vi "RT_Control_Adrian_AllIncluded.vi"(10 "rt fifo":refnum<k33>, 11 "Parameters":T1) -> (0 "error out":errorcluster, 2 "Delayed Cycles":dbl)   [LabVIEW 2021]
uses:
  parametersRT.ctl
  <vilib>/DAQmx/write.llb/DAQmx Write (Analog 1D DBL NChan 1Samp).vi
  <vilib>/DAQmx/read.llb/DAQmx Read (Analog 1D DBL NChan 1Samp).vi
  <vilib>/DAQmx/read.llb/DAQmx Read (Digital 2D U32 NChan NSamp).vi
  <vilib>/Analysis/baseanly.llb/Mean (DBL).vi
  <vilib>/DAQmx/configure/timing.llb/DAQmx Timing (Sample Clock).vi
  <vilib>/DAQmx/miscellaneous.llb/DAQmx Fill In Error Info.vi
  <resource>/objmgr/daqmx.rc
  <vilib>/Analysis/NI_AALBase.lvlib
panel:
  out "error out 7":errorcluster
  out "error out 6":errorcluster
  out "error out 5":errorcluster
  out "error out 4":errorcluster
  out "error out 3":errorcluster
  out "error out 2":errorcluster
  out "FB Raw Readings":dbl[][](array[numeric])
  in  "Stop Loop":bool
  in  "System Information":enum32{"RT System"}(tab)
  in  "source":tag
  in  "source 2":tag
  in  "RT Data Monitoring":enum32{"Forces", "Angles", "Power", "Pressure"}(tab)
  out "Bias Voltages":dbl[][](array[numeric])=[[-0.0710179470114859, -0.17463349299050945, -0.11016159714741332, 0.026018829634351103, 0.12897648926553976, 0.08259620236774425]]
  out "Bias Vector":dbl[](array[numeric])=[-0.0710179470114859, -0.17463349299050945, -0.11016159714741332, 0.026018829634351103, 0.12897648926553976, 0.08259620236774425]
  in  "Bias":bool
  in  "Unbias":bool
  in  "Zero Angle  Offset":dbl[](array[numeric])=[8.53, -8.09, 79.37, 29.36]
  # "Important! Set angle offset before reading angles"
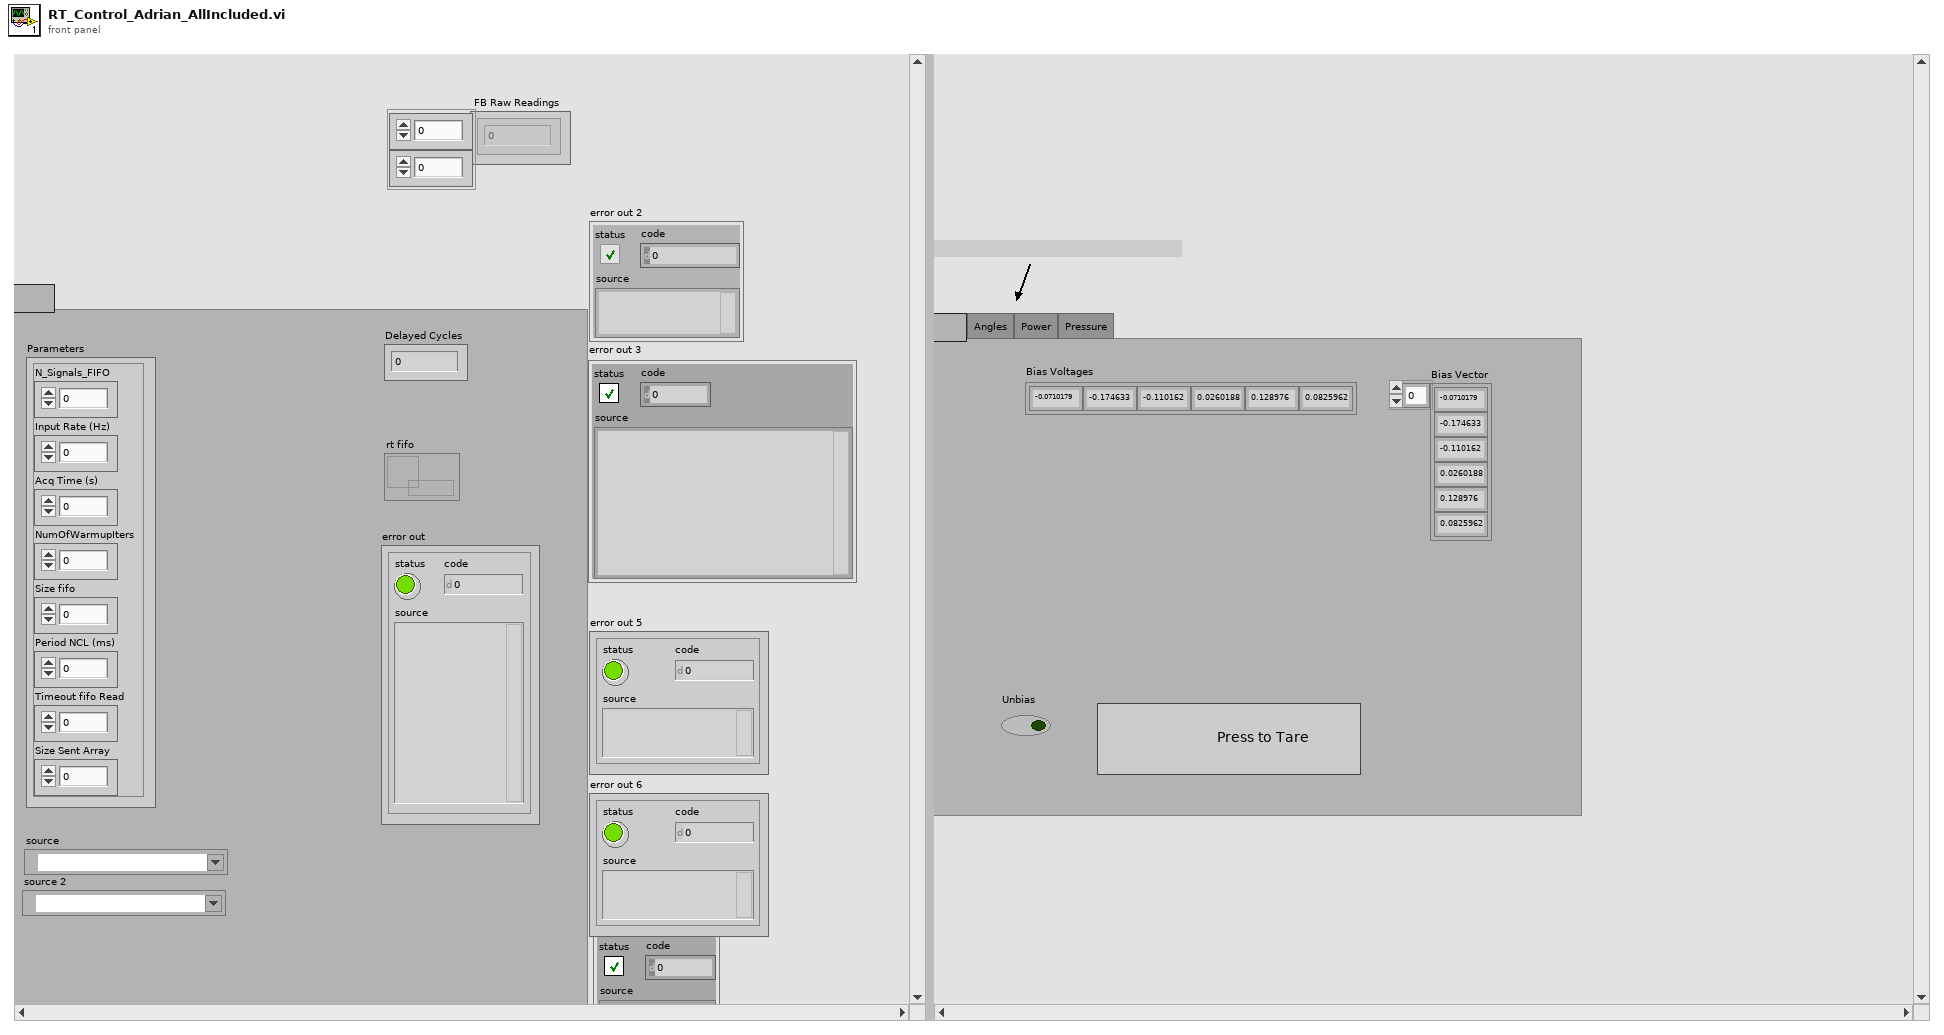
[diagram p1: front panel]
types:
  T1 = typedef "parametersRT.ctl" = cluster{"N_Signals_FIFO":u32, "Input Rate (Hz)":dbl, "Acq Time (s)":dbl, "NumOfWarmupIters":u32, "Size fifo":u32, "Period NCL (ms)":i64, "Timeout fifo Read":i32, "Size Sent Array":i32}
  T2 = cluster{"Csn task out":refnum<k21>, "CLK task out":refnum<k21>, "D0 task out":refnum<k21>}
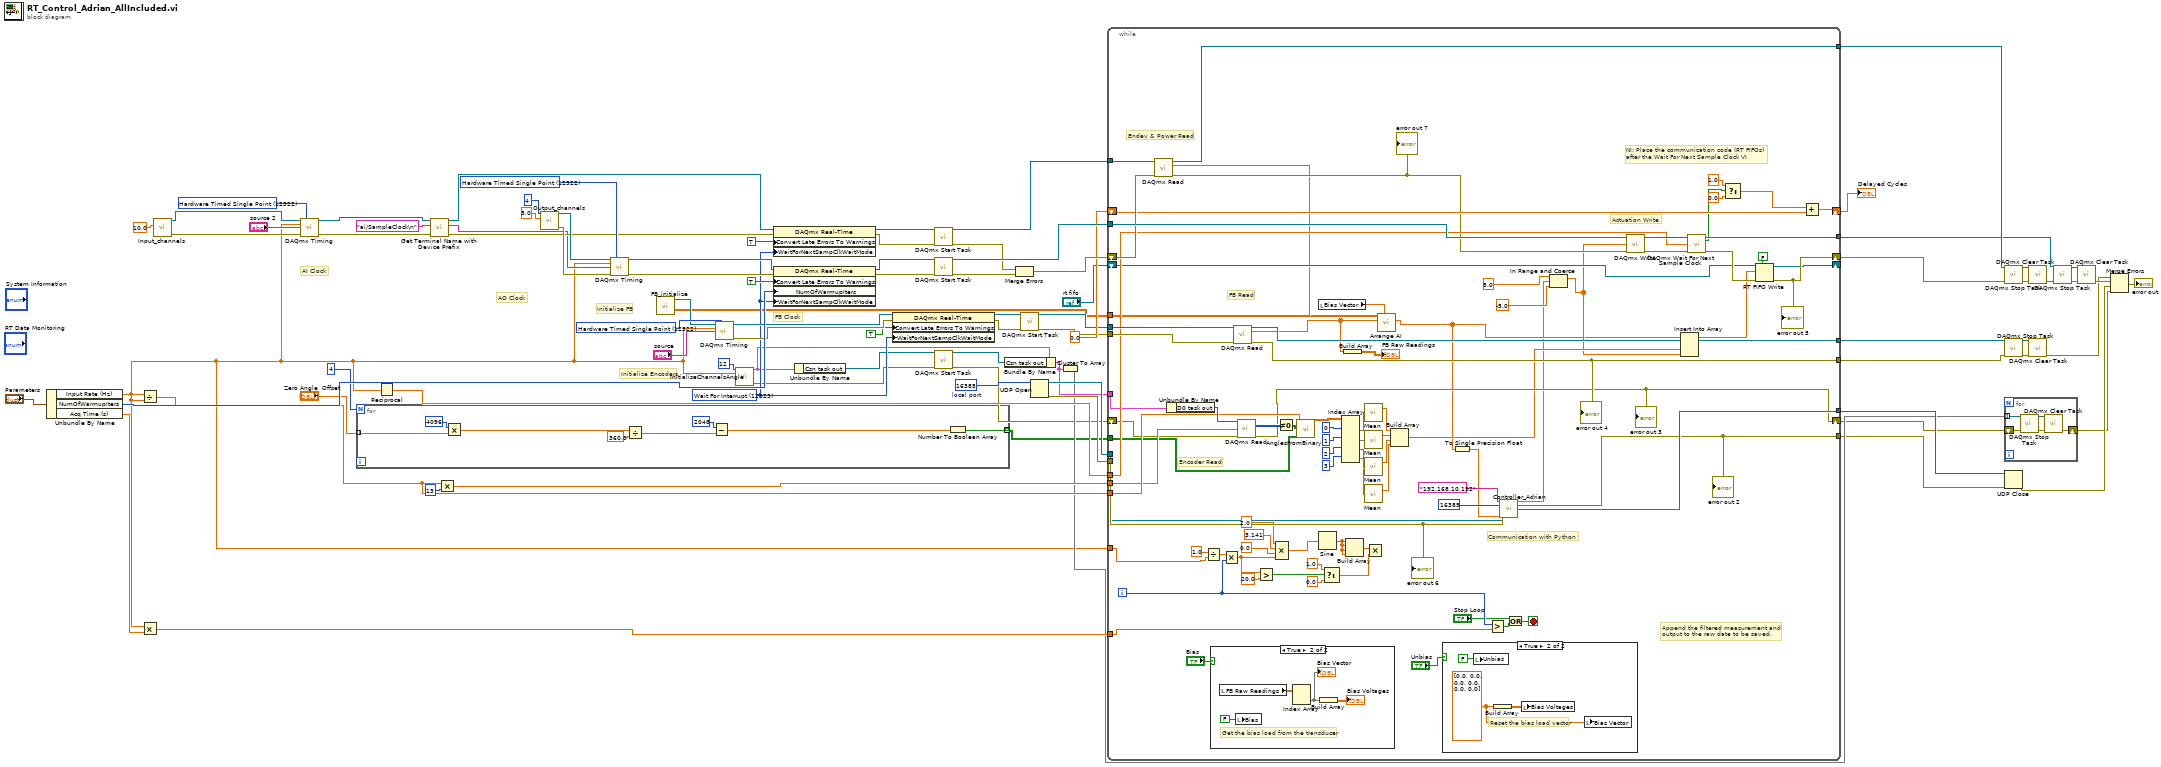
[diagram p0: block diagram]
diagram:
  w49 = 12522 items=["Finite Samples"=10178, "Continuous Samples"=10123, "Hardware Timed Single Point"=12522] ("sample mode")
  w59 = u16 16385  # local port
  w66 = 12522 items=["Finite Samples"=10178, "Continuous Samples"=10123, "Hardware Timed Single Point"=12522] ("sample mode")
  w44 = 12523 items=["Wait For Interrupt"=12523, "Poll"=12524, "Yield"=12525] ("WaitForNextSampClkWaitMode")
  w86 = 12522 items=["Finite Samples"=10178, "Continuous Samples"=10123, "Hardware Timed Single Point"=12522] ("sample mode")
  # "Initialize Encoders"
  # "Initialize FB"
  # "AO Clock"
  # "AI Clock"
  # "FB Clock"
  n1 = Unbundle By Name("Parameters") -> ("Input Rate (Hz)"=w1:dbl, "NumOfWarmupIters"=w73:u32, "Acq Time (s)"=w80:dbl)
  n2 = Divide(x=w1, y=w1) -> (x/y=w11:dbl)
  n3 = Multiply(x=w1, y=w80) -> (x*y=w54:dbl)
  n4 = call "Input_channels.vi"("Range"=10.0) -> ("error out"=w68:errorcluster, "Refnum out"=w67:refnum<k21>)  [unwired: 9 in]
  n5 = call-poly <vilib>:"DAQmx Timing.vi"("task/channels in"=w67, "sample mode"=w66, "rate"=w1, "source"="source 2", "error in"=w68) -> ("task out"=w37:refnum<k21>, "error out"=w35:errorcluster)  [unwired: 9 in]
  n6 = for {
    N: 4 -> [_]
    tunnel: [w91] -> w3 mode=indexing
    tunnel: "Zero Angle  Offset" -> [w94] mode=indexing
    n7 = Multiply(x=4096, y=w94) -> (x*y=w95:dbl)
    n8 = Divide(x=w95, y=360.0) -> (x/y=w89:dbl)
    n9 = Subtract(x=2048, y=w89) -> (x-y=w88:dbl)
    n10 = Number To Boolean Array(number=w88) -> (Boolean array=w91:bool[])
  }
  n11 = Reciprocal(x=w1) -> (1/x=w85:dbl)
  n12 = call "Get Terminal Name with Device Prefix.vi"("error in (no error)"=w35, "Local Terminal Name"="ai/SampleClock\n", "task/channels in"=w37) -> ("error out"=w34:errorcluster, "Terminal Name with Device Prefix"=w33:tag, "task out"=w36:refnum<k21>)  [unwired: 6 in]
  n13 = Multiply(x=w11, y=13) -> (x*y=w9:dbl)
  n14 = call "Output_channels.vi"("Range"=5.0 ("Maximum Value"), "nchan"=4) -> ("error out"=w77:errorcluster, "Refnum out"=w76:refnum<k21>)  [unwired: 8 in]
  n15 = call-poly <vilib>:"DAQmx Timing.vi"("task/channels in"=w76, "sample mode"=w86, "rate"=w1, "source"=w33, "error in"=w77) -> ("task out"=w84:refnum<k21>, "error out"=w83:errorcluster)  [unwired: 9 in]
  n16 = call "FB_initialize.vi"() -> ("Transformed Calibration Matrix"=w41:dbl[][], "FB out"=w45:refnum<k21>)  [unwired: 9 in, 1 out]
  n17 = call-poly <vilib>:"DAQmx Timing.vi"("task/channels in"=w45, "sample mode"=w49, "rate"=w1, "source"="source") -> ("task out"=w51:refnum<k21>, "error out"=w50:errorcluster)  [unwired: 10 in]
  n18 = call "InitialiseChannelsAngle.vi"("Number of data bits"=12, "Fs"=w1) -> ("output cluster"=w12:T2, "error out"=w13:errorcluster)  [unwired: 12 in]
  n19 = property class="DAQmx Real-Time"(reference=w36, error in=w34, "Convert Late Errors To Warnings"=TRUE, "WaitForNextSampClkWaitMode"=w44) -> (reference out=w63:refnum<k21>, error out=w62:errorcluster)
  n20 = property class="DAQmx Real-Time"(reference=w84, error in=w83, "Convert Late Errors To Warnings"=TRUE, "NumOfWarmupIters"=w73, "WaitForNextSampClkWaitMode"=w44) -> (reference out=w81:refnum<k21>, error out=w70:errorcluster)
  n21 = Unbundle By Name(w12) -> ("Csn task out"=w17:refnum<k21>)
  n22 = property class="DAQmx Real-Time"(reference=w51, error in=w50, "Convert Late Errors To Warnings"=TRUE ("ConvLateErrorsToWarnings"), "WaitForNextSampClkWaitMode"=w44) -> (reference out=w46:refnum<k21>, error out=w47:errorcluster)
  n23 = call <vilib>:"DAQmx Start Task.vi"("task/channels in"=w63, "error in"=w62) -> ("task out"=w79:refnum<k21>, "error out"=w61:errorcluster)  [unwired: 12 in]
  n24 = call <vilib>:"DAQmx Start Task.vi"("task/channels in"=w81, "error in"=w70) -> ("task out"=w78:refnum<k21>, "error out"=w69:errorcluster)  [unwired: 12 in]
  n25 = call <vilib>:"DAQmx Start Task.vi"("task/channels in"=w17, "error in"=w13) -> ("task out"=w16:refnum<k21>, "error out"=w6:errorcluster)  [unwired: 12 in]
  n26 = Bundle By Name(cluster=w12, "Csn task out"=w16) -> (w10:T2)
  n27 = Merge Errors(w61, w69) -> (w60:errorcluster)
  n28 = call <vilib>:"DAQmx Start Task.vi"("task/channels in"=w46, "error in"=w47) -> ("task out"=w43:refnum<k21>, "error out"=w42:errorcluster)  [unwired: 12 in]
  n29 = UDP Open(11:w59) -> (port=w57:refnum<k16>, 0:w58:errorcluster)  [unwired: 4 in, 1 out]
  n30 = Cluster To Array(cluster=w10) -> (array=w8:refnum<k21>[])
  n31 = while {
    shift-right: [w134] -> w26
    shift-left: w60 -> [w174]
    shift-right: [w179] -> w87
    shift-left: 0.0 ("f") -> [w168]
    tunnel: w85 -> [w157]
    tunnel: w54 -> [w178]
    tunnel: w78 -> [w177]
    tunnel: [w175] -> w25
    tunnel: w79 -> [w176]
    tunnel: [w159] -> w21
    tunnel: w58 -> [w173]
    tunnel: w57 -> [w172]
    tunnel: [w171] -> w56
    tunnel: w43 -> [w167]
    tunnel: w42 -> [w166]
    tunnel: w41 -> [w106]
    tunnel: [w163] -> w31
    tunnel: [w162] -> w29
    tunnel: w11 -> [w140]
    tunnel: w10 -> [w139]
    tunnel: w9 -> [w138]
    shift-right: [w137] -> w7
    shift-left: w6 -> [w136]
    shift-right: [w132] -> _
    shift-left: "rt fifo" -> [w131]
    tunnel: w3 -> [w114]
    tunnel: [w113] -> w2
    tunnel: w1 -> [w112]
    i -> [w125]
    stop <- w109 stop-if-true
    # "NI: Place the communication code (RT FIFOs) \nafter the Wait For Next Sample Clock VI"
    # "Communication with Python"
    # "Actuation Write"
    # "Encoder Read"
    # "Endev & Power Read"
    # "FB Read"
    # "Append the filtered measurement and \noutput to the raw date to be saved."
    n32 = call-poly <vilib>:"DAQmx Read.vi"("task/channels in"=w176, "error in"=w174) -> ("task out"=w175:refnum<k21>, "data"=w108:dbl[], "error out"=w129:errorcluster)  [unwired: 11 in]
    "error out 7" <- w129
    n33 = Unbundle By Name(w139) -> ("D0 task out"=w156:refnum<k21>)
    n34 = Divide(x=1.0, y=w112) -> (x/y=w123:dbl)
    n35 = case shown="True" "Bias" {
      frame False {
      }
      frame True {
        # "Get the bias load from the transducer"
        n36 = local read "FB Raw Readings"() -> (w189:dbl[][])
        n37 = local write "Bias"(FALSE) -> ()
        n38 = Index Array(array=w189) -> (element=w186:dbl[])  [unwired: 2 in]
        "Bias Vector" <- w186
        n39 = Build Array(w186) -> (→"Bias Voltages":dbl[][])
      }
    }
    n40 = Multiply(x=w123, y=w125) -> (x*y=w119:dbl)
    n41 = call-poly <vilib>:"DAQmx Read.vi"("task/channels in"=w167, "error in"=w166) -> ("task out"=w163:refnum<k21>, "data"=w103:dbl[], "error out"=w162:errorcluster)  [unwired: 11 in]
    "error out 4" <- w162
    n42 = call-poly <vilib>:"DAQmx Read.vi"("task/channels in"=w156, "number of samples per channel"=w138, "error in"=w136) -> ("data"=w155:u32[][], "error out"=w137:errorcluster)  [unwired: 10 in, 1 out]
    "error out 3" <- w137
    n43 = Greater?(x=w119, y=20.0) -> (0:w115:bool)
    n44 = Compound Arithmetic op=MULTIPLY(2.0 ("value"), 3.141 ("value"), 0.0 ("value"), w119) -> (w122:dbl)
    n45 = Not Equal To 0?(x=w155) -> (x != 0?=w141:bool[][])
    n46 = call "AnglesFromBinary.vi"("Binary Offset"=w114, "Array"=w141, "Buffer Length"=w140) -> ("Unwrapped Phase"=w154:dbl[][])  [unwired: 8 in]
    n47 = local read "Bias Vector"() -> (w107:dbl[])
    n48 = Sine(x=w122) -> (sin(x)=w121:dbl)
    n49 = Select(t=1.0, s=w115, f=0.0) -> (s? t:f=w105:dbl)
    n50 = Index Array(array=w154, index (row) #1=0 ("index (row)"), index (row) #2=1 ("index (row)"), index (row) #3=2 ("index (row)"), index (row) #4=3 ("index (row)")) -> (element #1=w149:dbl[], element #2=w148:dbl[], element #3=w147:dbl[], element #4=w146:dbl[])  [unwired: 4 in]
    n51 = Build Array(w103) -> (→"FB Raw Readings":dbl[][])
    n52 = Build Array(w121, w121, w121, w121) -> (w120:dbl[])
    n53 = call-poly <vilib>:"Mean.vi"("X"=w149) -> ("mean"=w142:dbl)  [unwired: 1 out]
    n54 = call-poly <vilib>:"Mean.vi"("X"=w148) -> ("mean"=w143:dbl)  [unwired: 1 out]
    n55 = call-poly <vilib>:"Mean.vi"("X"=w147) -> ("mean"=w144:dbl)  [unwired: 1 out]
    n56 = call-poly <vilib>:"Mean.vi"("X"=w146) -> ("mean"=w145:dbl)  [unwired: 1 out]
    n57 = Multiply(x=w120, y=w105) -> ()  [unwired: 1 out]
    n58 = call "Arrange AI.vi"("Transformed Calibration Matrix"=w106, "Bias Vector"=w107, "FB data"=w103, "EDV + Voltage data"=w108) -> ("FIFO Data (7EDV+3Force+4Power+4Voltage)"=w97:dbl[])  [unwired: 6 in, 1 out]
    n59 = Build Array(w142, w143, w144, w145) -> (w104:dbl[])
    n60 = case shown="True" "Unbias" {
      frame False {
      }
      frame True {
        w184 = dbl[] [0.0, 0.0, 0.0, 0.0, 0.0, 0.0]
        # "Reset the bias load vector"
        n61 = local write "Unbias"(FALSE) -> ()
        n62 = Build Array(w184) -> (w183:dbl[][])
        n63 = local write "Bias Voltages"(w183) -> ()
        n64 = local write "Bias Vector"(w184) -> ()
      }
    }
    n65 = To Single Precision Float(number=w97) -> (single precision float=w98:sgl[])
    n66 = Greater?(x=w125, y=w178) -> (0:w110:bool)
    n67 = call "Controller_Adrian.vi"("name 2"="192.168.10.192", "port or service name"=u16 16389, "connection ID"=w172, "error in (no error)"=w173, "x"=w98) -> ("*(type *) &x"=w96:dbl[], "error out"=w113:errorcluster, "connection ID out"=w171:refnum<k16>)  [unwired: 8 in]
    "error out 2" <- w113
    n68 = Or(x="Stop Loop", y=w110) -> (x .or. y?=w109:bool)
    n69 = In Range and Coerce(upper limit=5.0, x=w96, lower limit=-5.0) -> (coerced(x)=w101:dbl[])  [unwired: 1 out]
    n70 = call-poly <vilib>:"DAQmx Write.vi"("task/channels in"=w177, "data"=w101, "error in"=w129) -> ("task out"=w160:refnum<k21>, "error out"=w161:errorcluster)  [unwired: 10 in, 1 out]
    n71 = Insert Into Array(array=w97, new element #1=w104, new element #2=w101) -> (w130:dbl[])  [unwired: 1 in]
    n72 = call <vilib>:"DAQmx Wait For Next Sample Clock.vi"("task/channels in"=w160, "timeout (sec)"=w157, "error in"=w161) -> ("task out"=w159:refnum<k21>, "is late?"=w158:bool, "error out"=w133:errorcluster)  [unwired: 10 in]
    n73 = Select(t=1.0, s=w158, f=0.0) -> (s? t:f=w180:dbl)
    n74 = RT FIFO Write(0:w131, 1:w130, 3:w133, 5:FALSE ("overwrite on timeout (T)")) -> (8:w132:refnum<k33>, 11:w134:errorcluster)  [unwired: 1 in, 2 out]
    "error out 5" <- w134
    n75 = Add(x=w180, y=w168) -> (x+y=w179:dbl)
    "error out 6" <- w173
  }
  "Delayed Cycles" <- w87
  n76 = call <vilib>:"DAQmx Stop Task.vi"("task/channels in"=w25, "error in"=w26) -> ("task out"=w24:refnum<k21>, "error out"=w27:errorcluster)  [unwired: 12 in]
  n77 = call <vilib>:"DAQmx Stop Task.vi"("task/channels in"=w31, "error in"=w29) -> ("task out"=w30:refnum<k21>, "error out"=w28:errorcluster)  [unwired: 12 in]
  n78 = for {
    tunnel: w8 -> [w194] mode=indexing
    shift-right: [w190] -> w5
    shift-left: w7 -> [w192]
    n79 = call <vilib>:"DAQmx Stop Task.vi"("task/channels in"=w194, "error in"=w192) -> ("task out"=w193:refnum<k21>, "error out"=w191:errorcluster)  [unwired: 12 in]
    n80 = call <vilib>:"DAQmx Clear Task.vi"("task in"=w193, "error in"=w191) -> ("error out"=w190:errorcluster)  [unwired: 13 in]
  }
  n81 = UDP Close(connection ID=w56, 8:w2) -> (error out=w55:errorcluster)  [unwired: 1 out]
  n82 = call <vilib>:"DAQmx Clear Task.vi"("task in"=w24, "error in"=w27) -> ("error out"=w23:errorcluster)  [unwired: 13 in]
  n83 = call <vilib>:"DAQmx Clear Task.vi"("task in"=w30, "error in"=w28) -> ("error out"=w40:errorcluster)  [unwired: 13 in]
  n84 = call <vilib>:"DAQmx Stop Task.vi"("task/channels in"=w21, "error in"=w23) -> ("task out"=w20:refnum<k21>, "error out"=w22:errorcluster)  [unwired: 12 in]
  n85 = call <vilib>:"DAQmx Clear Task.vi"("task in"=w20, "error in"=w22) -> ("error out"=w72:errorcluster)  [unwired: 13 in]
  n86 = Merge Errors(w40, w72, w55, w5) -> (→"error out":errorcluster)
